vi "configwave.vi"() -> ()   [LabVIEW 2017]
panel:
  in  "Configurações da Onda":T1
  out "output cluster":T2
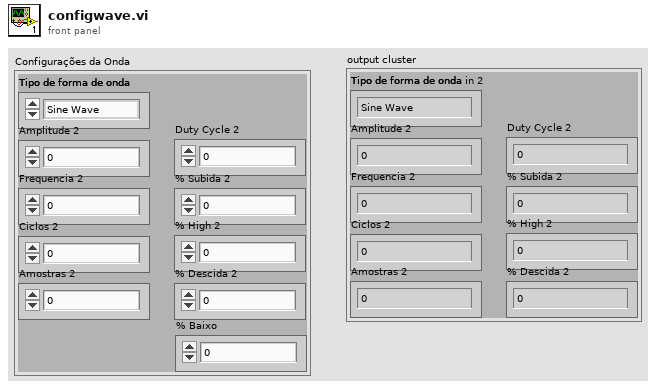
[diagram p1: front panel]
types:
  T1 = cluster{"Tipo de forma de onda ":enum16{"Sine Wave", "Triangle Wave", "Square Wave", "Sawtooth Wave", "Trapezoidal Wave"}, "Amplitude 2":dbl, "Frequencia 2":dbl, "Ciclos 2":dbl, "Duty Cycle 2":dbl, "% Subida 2":dbl, "% High 2":dbl, "% Descida 2":dbl, "Amostras 2":dbl, "% Baixo":dbl}
  T2 = cluster{"Tipo de forma de onda in 2":enum16{"Sine Wave", "Triangle Wave", "Square Wave", "Sawtooth Wave", "Trapezoidal Wave"}, "Amplitude 2":dbl, "Frequencia 2":dbl, "Ciclos 2":dbl, "Duty Cycle 2":dbl, "% Subida 2":dbl, "% High 2":dbl, "% Descida 2":dbl, "Amostras 2":dbl}
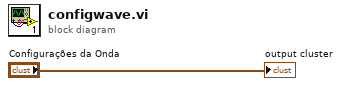
[diagram p0: block diagram]
diagram:
  "output cluster" <- "Configurações da Onda"
